vi "Logger_simple.vi"(0 "Name":string="Example.txt", 1 "Relative path":string="Example.txt", 2 "Desired logging-Frequency [Hz]":dbl=3.0, 3 "error in":errorcluster) -> (6 "Filename Out":path, 9 "error out":errorcluster)   [LabVIEW 2013]
doc: "Logs the Data fed to it by shared variables at the desired frequency."
uses:
  IMU/IMU_Data_Type_Def.ctl
  <vilib>/Utility/file.llb/Write To Spreadsheet File (DBL).vi
panel:
  out "Less then 25Hz":bool
  out "Elapsed Time":u32
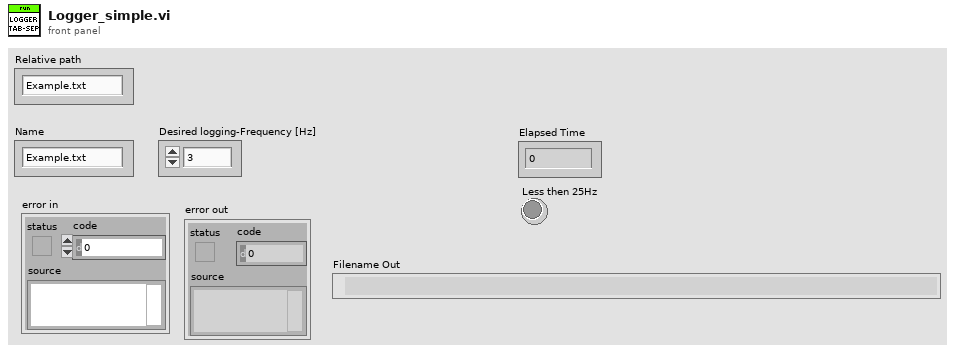
[diagram p1: front panel]
types:
  T1 = typedef "IMU_Data_Type_Def.ctl" = cluster{timestamp, "X_Gyro_Out":dbl, "Y_Gyro_Out":dbl, "Z_Gyro_Out":dbl, "X_Accl_Out":dbl, "Y_Accl_Out":dbl, "Z_Accl_Out":dbl, "X_Magn_Out":dbl, "Y_Magn_Out":dbl, "Z_Magn_Out":dbl, "Temp_Out":dbl, "Barom_Out":dbl}
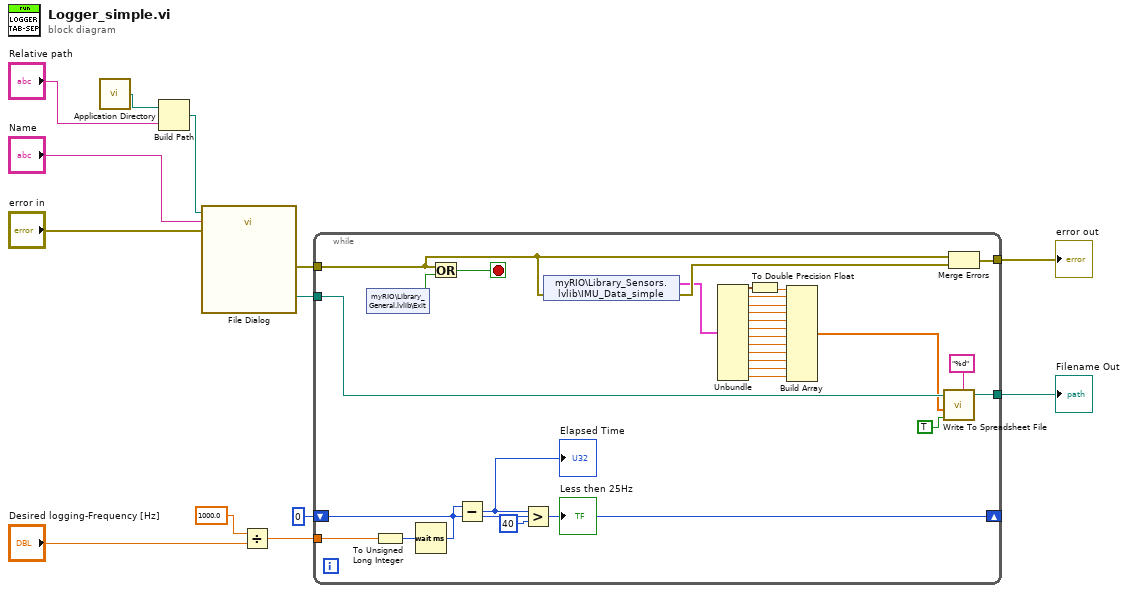
[diagram p0: block diagram]
diagram:
  n1 = call <vilib>:"Application Directory.vi"() -> ("Application Directory"=w4:path)
  n2 = Build Path(base path=w4, name or relative path="Relative path") -> (appended path=w2:path)
  n3 = call "File Dialog"("start path"=w2, "default name"="Name", "error in"="error in") -> ("selected path"=w10:path, "error out"=w12:errorcluster)  [unwired: 9 in, 2 out]
  n4 = Divide(x=1000.0, y="Desired logging-Frequency [Hz]") -> (x/y=w6:dbl)
  n5 = while {
    shift-right: [w38] -> _
    shift-left: u32 0 ("millisecond timer value") -> [w43]
    tunnel: w12 -> [w30]
    tunnel: [w32] -> w11
    tunnel: w10 -> [w40]
    tunnel: [w39] -> w9
    tunnel: w6 -> [w33]
    stop <- w42 stop-if-true
    n6 = shared-variable "myRIO\\Library_General.lvlib\\Exit"() -> (w44:bool)  [unwired: 1 in, 1 out]
    n7 = To Unsigned Long Integer(number=w33) -> (unsigned 32bit integer=w34:u32)
    n8 = Wait (ms)(milliseconds to wait=w34) -> (millisecond timer value=w38:u32)
    n9 = Or(x=w30, y=w44) -> (x .or. y?=w42:bool)
    n10 = Subtract(x=w38, y=w43) -> (x-y=w37:u32)
    "Elapsed Time" <- w37
    n11 = Greater?(x=w37, y=u32 40) -> (0:→"Less then 25Hz":bool)
    n12 = shared-variable "myRIO\\Library_Sensors.lvlib\\IMU_Data_simple"(error in=w30) -> (w29:T1, error out=w31:errorcluster)
    n13 = Unbundle(w29) -> (w16:timestamp, "X_Gyro_Out"=w28:dbl, "Y_Gyro_Out"=w27:dbl, "Z_Gyro_Out"=w26:dbl, "X_Accl_Out"=w25:dbl, "Y_Accl_Out"=w24:dbl, "Z_Accl_Out"=w23:dbl, "X_Magn_Out"=w22:dbl, "Y_Magn_Out"=w21:dbl, "Z_Magn_Out"=w20:dbl, "Temp_Out"=w19:dbl, "Barom_Out"=w18:dbl)
    n14 = To Double Precision Float(number=w16) -> (double precision float=w15:dbl)
    n15 = Build Array(w15, w28, w27, w26, w25, w24, w23, w22, w21, w20, w19, w18) -> (w14:dbl[])
    n16 = call-poly <vilib>:"Write To Spreadsheet File.vi"("format (%.3f)"="%d", "append to file? (new file:F)"=TRUE, "1D data"=w14, "file path (dialog if empty)"=w40) -> ("new file path (Not A Path if cancelled)"=w39:path)  [unwired: 4 in]
    n17 = Merge Errors(w30, w31) -> (w32:errorcluster)
  }
  "error out" <- w11
  "Filename Out" <- w9
